vi "subViFormulaGenerator_8channel.vi"(2 "sampling info":cluster{"Fs":dbl, "#s":dbl}={"Fs"=1000.0, "#s"=1000.0} {"Fs" format="%.2p"}, 3 "error in (no error)":errorcluster, 4 "formular in":T1(array[cluster]), 5 "regulatorArray":cluster{"offset":dbl, "scale":dbl}[](array[cluster]) {"scale" format="%0.2f"; "offset" format="%0.2p"}) -> (0 "error out":errorcluster, 1 "formular out":waveform(dbl)[](array[waveform]))   [LabVIEW 2021]
panel:
  # "子程序，将之前的4段函数整合到8个通道中"
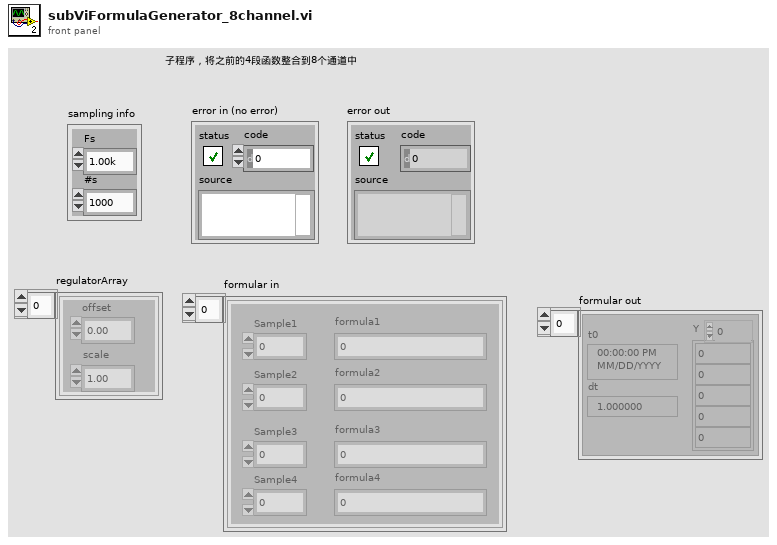
[diagram p1: front panel]
types:
  T1 = cluster{"Sample1":dbl, "formula1":string, "Sample2":dbl, "formula2":string, "Sample3":dbl, "formula3":string, "Sample4":dbl, "formula4":string}[]
  T2 = cluster{"formular in[0]":cluster{"Sample1":dbl, "formula1":string, "Sample2":dbl, "formula2":string, "Sample3":dbl, "formula3":string, "Sample4":dbl, "formula4":string}, "formular in[1]":cluster{"Sample1":dbl, "formula1":string, "Sample2":dbl, "formula2":string, "Sample3":dbl, "formula3":string, "Sample4":dbl, "formula4":string}, "formular in[2]":cluster{"Sample1":dbl, "formula1":string, "Sample2":dbl, "formula2":string, "Sample3":dbl, "formula3":string, "Sample4":dbl, "formula4":string}, "formular in[3]":cluster{"Sample1":dbl, "formula1":string, "Sample2":dbl, "formula2":string, "Sample3":dbl, "formula3":string, "Sample4":dbl, "formula4":string}, "formular in[4]":cluster{"Sample1":dbl, "formula1":string, "Sample2":dbl, "formula2":string, "Sample3":dbl, "formula3":string, "Sample4":dbl, "formula4":string}, "formular in[5]":cluster{"Sample1":dbl, "formula1":string, "Sample2":dbl, "formula2":string, "Sample3":dbl, "formula3":string, "Sample4":dbl, "formula4":string}, "formular in[6]":cluster{"Sample1":dbl, "formula1":string, "Sample2":dbl, "formula2":string, "Sample3":dbl, "formula3":string, "Sample4":dbl, "formula4":string}, "formular in[7]":cluster{"Sample1":dbl, "formula1":string, "Sample2":dbl, "formula2":string, "Sample3":dbl, "formula3":string, "Sample4":dbl, "formula4":string}, "formular in[8]":cluster{"Sample1":dbl, "formula1":string, "Sample2":dbl, "formula2":string, "Sample3":dbl, "formula3":string, "Sample4":dbl, "formula4":string}}
  T3 = cluster{"regulatorArray[0]":cluster{"offset":dbl, "scale":dbl}, "regulatorArray[1]":cluster{"offset":dbl, "scale":dbl}, "regulatorArray[2]":cluster{"offset":dbl, "scale":dbl}, "regulatorArray[3]":cluster{"offset":dbl, "scale":dbl}, "regulatorArray[4]":cluster{"offset":dbl, "scale":dbl}, "regulatorArray[5]":cluster{"offset":dbl, "scale":dbl}, "regulatorArray[6]":cluster{"offset":dbl, "scale":dbl}, "regulatorArray[7]":cluster{"offset":dbl, "scale":dbl}, "regulatorArray[8]":cluster{"offset":dbl, "scale":dbl}}
  T4 = cluster{"Sample1":dbl, "formula1":string, "Sample2":dbl, "formula2":string, "Sample3":dbl, "formula3":string, "Sample4":dbl, "formula4":string}
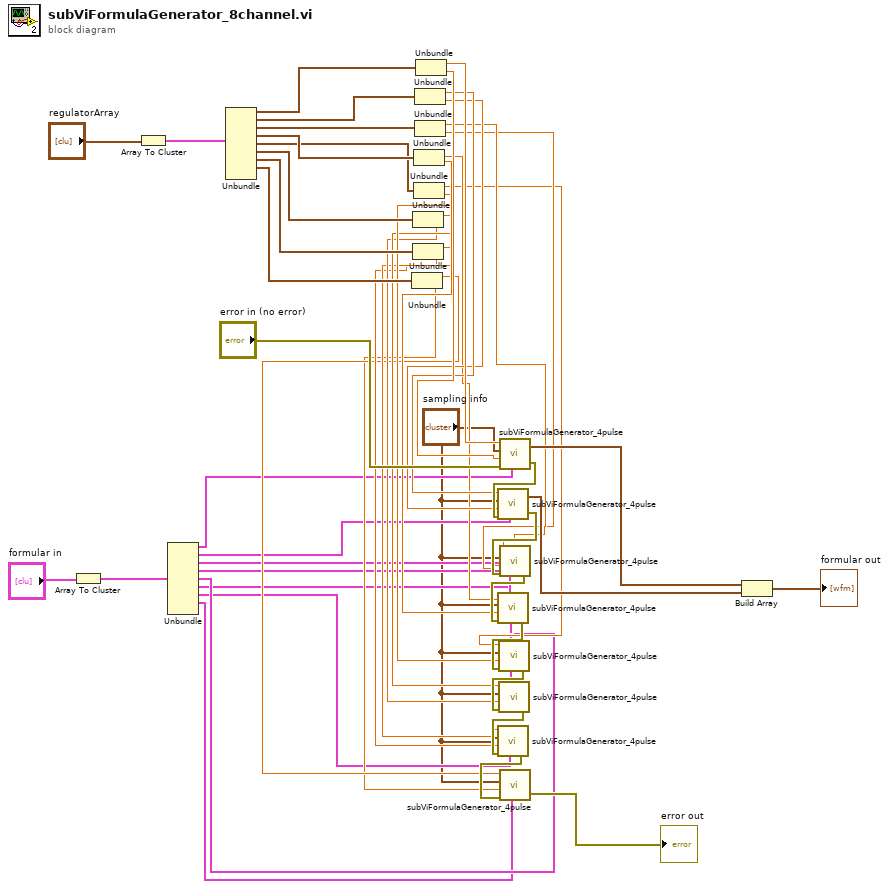
[diagram p0: block diagram]
diagram:
  n1 = Array To Cluster(array="formular in") -> (cluster=w37:T2)
  n2 = Array To Cluster(array="regulatorArray") -> (cluster=w34:T3)
  n3 = Unbundle "Unbundle"(w37) -> ("formular in[0]"=w9:T4, "formular in[1]"=w8:T4, "formular in[2]"=w7:T4, "formular in[3]"=w6:T4, "formular in[4]"=w5:T4, "formular in[5]"=w4:T4, "formular in[6]"=w3:T4, "formular in[7]"=w2:T4)  [unwired: 1 out]
  n4 = Unbundle(w34) -> ("regulatorArray[0]"=w33:cluster{"offset":dbl, "scale":dbl}, "regulatorArray[1]"=w32:cluster{"offset":dbl, "scale":dbl}, "regulatorArray[2]"=w31:cluster{"offset":dbl, "scale":dbl}, "regulatorArray[3]"=w30:cluster{"offset":dbl, "scale":dbl}, "regulatorArray[4]"=w29:cluster{"offset":dbl, "scale":dbl}, "regulatorArray[5]"=w28:cluster{"offset":dbl, "scale":dbl}, "regulatorArray[6]"=w27:cluster{"offset":dbl, "scale":dbl}, "regulatorArray[7]"=w26:cluster{"offset":dbl, "scale":dbl})  [unwired: 1 out]
  n5 = Unbundle(w26) -> ("offset"=w11:dbl, "scale"=w10:dbl)
  n6 = Unbundle(w28) -> ("offset"=w15:dbl, "scale"=w14:dbl)
  n7 = Unbundle(w27) -> ("offset"=w13:dbl, "scale"=w12:dbl)
  n8 = Unbundle(w30) -> ("offset"=w19:dbl, "scale"=w18:dbl)
  n9 = Unbundle(w29) -> ("offset"=w17:dbl, "scale"=w16:dbl)
  n10 = Unbundle(w32) -> ("offset"=w23:dbl, "scale"=w22:dbl)
  n11 = Unbundle(w31) -> ("offset"=w21:dbl, "scale"=w20:dbl)
  n12 = Unbundle(w33) -> ("offset"=w25:dbl, "scale"=w24:dbl)
  n13 = call "subViFormulaGenerator_4pulse.vi"("offset"=w25, "sampling info"="sampling info", "scale"=w24, "error in (no error)"="error in (no error)", "functionInfo"=w9) -> ("waveform out"=w42:waveform(dbl), "error out"=w49:errorcluster)
  n14 = call "subViFormulaGenerator_4pulse.vi"("offset"=w23, "sampling info"="sampling info", "scale"=w22, "error in (no error)"=w49, "functionInfo"=w8) -> ("waveform out"=w41:waveform(dbl), "error out"=w48:errorcluster)
  n15 = call "subViFormulaGenerator_4pulse.vi"("offset"=w21, "sampling info"="sampling info", "scale"=w20, "error in (no error)"=w48, "functionInfo"=w7) -> ("error out"=w47:errorcluster)  [unwired: 1 out]
  n16 = call "subViFormulaGenerator_4pulse.vi"("offset"=w19, "sampling info"="sampling info", "scale"=w18, "error in (no error)"=w47, "functionInfo"=w6) -> ("error out"=w46:errorcluster)  [unwired: 1 out]
  n17 = call "subViFormulaGenerator_4pulse.vi"("offset"=w17, "sampling info"="sampling info", "scale"=w16, "error in (no error)"=w46, "functionInfo"=w5) -> ("error out"=w45:errorcluster)  [unwired: 1 out]
  n18 = call "subViFormulaGenerator_4pulse.vi"("offset"=w15, "sampling info"="sampling info", "scale"=w14, "error in (no error)"=w45, "functionInfo"=w4) -> ("error out"=w44:errorcluster)  [unwired: 1 out]
  n19 = call "subViFormulaGenerator_4pulse.vi"("offset"=w13, "sampling info"="sampling info", "scale"=w12, "error in (no error)"=w44, "functionInfo"=w3) -> ("error out"=w43:errorcluster)  [unwired: 1 out]
  n20 = call "subViFormulaGenerator_4pulse.vi"("offset"=w11, "sampling info"="sampling info", "scale"=w10, "error in (no error)"=w43, "functionInfo"=w2) -> ("error out"=→"error out":errorcluster)  [unwired: 1 out]
  n21 = Build Array(w42, w41) -> (→"formular out":waveform(dbl)[])
